vi "Get Log File Location.vi"(8 "error in (no error)":errorcluster, 11 "log file in":T1 format="%.0x") -> (0 "error out":errorcluster, 1 "timestamp file name":bool, 2 "directory parts":string[](array[string]), 3 "log file out":T1 format="%.0x", 4 "base file name":string, 5 "sample path":path)   [LabVIEW 2027, in "Embedded Data Logger Scripting.lvlib"]
uses:
  Embedded Data Logger Scripting.lvlib
  <vilib>/NI VeriStand/Custom Device API/Custom Device Item Ref.ctl
  Shared/Constants.vi
  <vilib>/NI VeriStand/Custom Device API/Get Item Property (String Array).vi
  <vilib>/NI VeriStand/Custom Device API/Get Item Property (Boolean).vi
  <vilib>/NI VeriStand/Custom Device API/Custom Device API.lvlib
  Shared/Embedded Data Logger Shared.lvlib
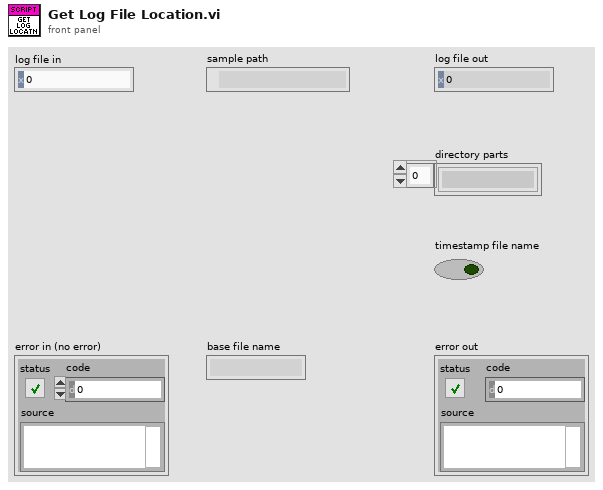
[diagram p1: front panel]
types:
  T1 = typedef "Custom Device API.lvlib/Custom Device Item Ref.ctl" = u64
  T2 = typedef "Custom Device API.lvlib/Custom Device Item Info.ctl" = cluster{"Name":string, "Is Channel":bool, "GUID":string, "Is Waveform":bool}
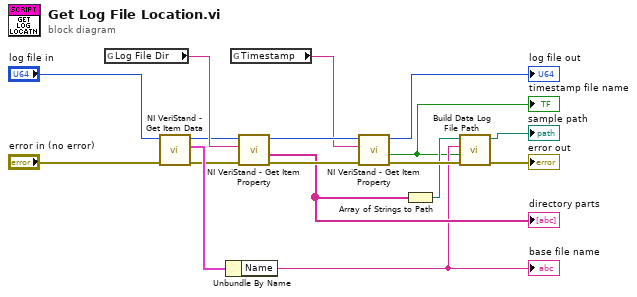
[diagram p0: block diagram]
diagram:
  n1 = global read "Constants.vi" "Log File Dir"() -> (w13:string)
  n2 = call <vilib>:"NI VeriStand - Get Item Data.vi"("error in (no error)"="error in (no error)", "Item Ref in"="log file in") -> ("error out"=w9:errorcluster, "Item Info"=w10:T2, "Item Ref out"=w8:T1)  [unwired: 7 out]
  n3 = Unbundle By Name(w10) -> ("Name"=w3:string)
  "base file name" <- w3
  n4 = global read "Constants.vi" "Timestamp"() -> (w14:string)
  n5 = call-poly <vilib>:"NI VeriStand - Get Item Property.vi"("error in (no error)"=w9, "Property Name"=w13, "Item Ref in"=w8) -> ("error out"=w16:errorcluster, "Value"=w5:string[], "Item Ref out"=w15:T1)  [unwired: 1 in, 5 out]
  "directory parts" <- w5
  n6 = call-poly <vilib>:"NI VeriStand - Get Item Property.vi"("error in (no error)"=w16, "Property Name"=w14, "Item Ref in"=w15) -> ("error out"=w7:errorcluster, "Value"=w2:bool, "Item Ref out"=→"log file out":T1)  [unwired: 1 in, 5 out]
  "timestamp file name" <- w2
  n7 = Array of Strings to Path(0:w5) -> (2:w4:path)  [unwired: 1 in]
  n8 = call "Build Data Log File Path.vi"("error in (no error)"=w7, "Timestamp"=w2, "Name"=w3, "Log File Directory"=w4) -> ("error out"=→"error out":errorcluster, "appended path"=→"sample path":path)  [unwired: 6 in]
